vi "Drive Controller.vi"(8 "error in":errorcluster) -> ()   [LabVIEW 2020]
doc: "This VI executes continuously carrying out the current operation and responding to updates or new operation requests. It will often contain the timing or control code that is difficult to place directly in TeleOp. This VI generally opens all sensors and motors and isolates the rest of the robot code from knowing implementation details of how the operations are carried out."
uses:
  <vilib>/Rock Robotics/WPI/Framework/Completion Status.ctl
  Drive Setpoints.ctl
  Drive Operations.ctl
  <vilib>/Rock Robotics/WPI/SafetyOutput/WPI_SafetyOutputConfigMenu.ctl
  <vilib>/Rock Robotics/WPI/RobotDrive/WPI_RobotDriveOpen2MotorWithExistingMotors.vi
  <vilib>/Rock Robotics/Network Tables/NT Write Numeric Array.vi
panel:
  in  "Interactive Values":T1
  in  "Buttons":cluster{"Execute Cmd":bool, "Abort Cmd":bool}
  out "Command Timing":cluster{"Start Time (ms)":u32, "Iterations":i32}
  out "Status":T3
  out "Setpoints":T4(graph)
  out "Current\nCmd":string
  # "Tip: The graph shows the motor setpoints. It may also be helpful to observe inputs and sensor values.\nYou may also want to display tuning or debugging controls."
  # "Interactive Command: You may fill in the settings for a command\nand schedule it with the Execute button. You can observe and abort\nany command while fine tuning the code for the controller."
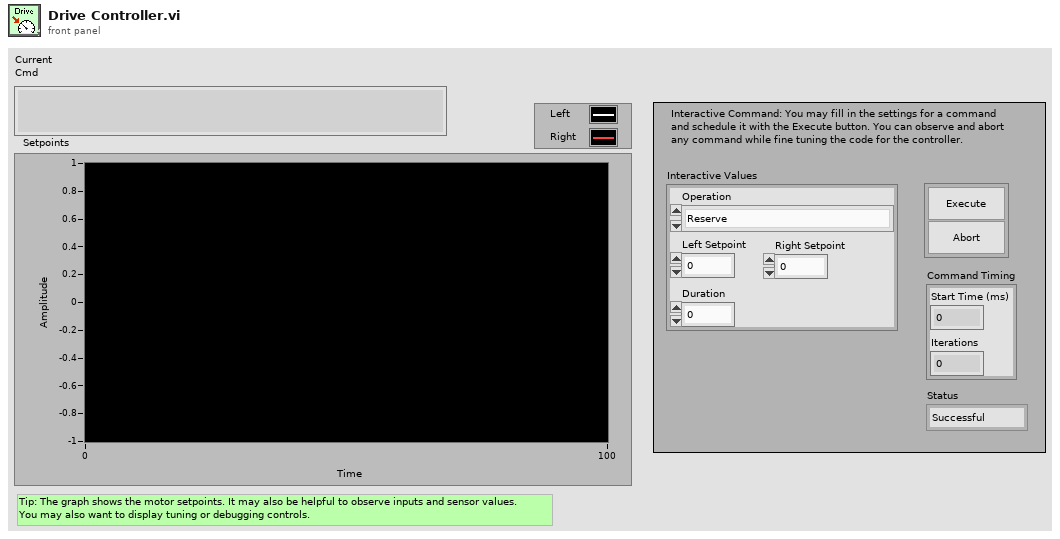
[diagram p1: front panel]
types:
  T1 = typedef "Drive Setpoints.ctl" = cluster{"Operation":T2, "Left Setpoint":dbl, "Right Setpoint":dbl, "Duration":dbl}
  T2 = typedef "Drive Operations.ctl" = enum16{"Reserve", "Read Current", "Immediate", "Drive for Time", "Drive for Distance"}
  T3 = typedef "Completion Status.ctl" = enum16{"Successful", "Aborted", "Incomplete"}
  T4 = cluster{"Left Setpoint":dbl, "Right Setpoint":dbl}
  T5 = typedef "WPI_SafetyOutputConfigMenu.ctl" = enum16{"Enable", "Disable"}
  T6 = typedef "WPI_MotorControlDeviceRef.ctl" = cluster{"DeviceStatus":errorcluster, "Type":T7, "PWM":cluster{"PWM Channel":T8, "DeadBand":T9}, "CAN":cluster{"Device Number":u8, "SetOutput VI Ref":variant, "GetOutput VI Ref":variant, "Enable VI Ref":variant, "Disable VI Ref":variant, "Data":variant}, "Invert":bool, "DIO PWM":cluster{"PWM \"Enable\" Channel":T8, "DIOChannel":T10, "PWM Rate":dbl}}
  T7 = typedef "WPI_MotorControlType.ctl" = enum16{"PWM", "CAN", "DIO PWM"}
  T8 = typedef "FPGA_DIOPWMChannel.ctl" = enum8{"PWM 0", "PWM 1", "PWM 2", "PWM 3", "PWM 4", "PWM 5", "PWM 6", "PWM 7", "PWM 8", "PWM 9", "PWM MXP 0", "PWM MXP 1", "PWM MXP 2", "PWM MXP 3", "PWM MXP 4", "PWM MXP 5", "PWM MXP 6", "PWM MXP 7", "PWM MXP 8", "PWM MXP 9", "Invalid"}
  T9 = typedef "WPI_PWMDeadband.ctl" = cluster{"Name":string, "maxPositivePwm":i32, "minPositivePwm":i32, "centerPwm":i32, "maxNegativePwm":i32, "minNegativePwm":i32, "angularRange":u16}
  T10 = typedef "FPGA_DIOChannel.ctl" = enum8{"DIO 0", "DIO 1", "DIO 2", "DIO 3", "DIO 4", "DIO 5", "DIO 6", "DIO 7", "DIO 8", "DIO 9", "DIO MXP 0", "DIO MXP 1", "DIO MXP 2", "DIO MXP 3", "DIO MXP 4", "DIO MXP 5", "DIO MXP 6", "DIO MXP 7", "DIO MXP 8", "DIO MXP 9", "DIO MXP 10", "DIO MXP 11", "DIO MXP 12", "DIO MXP 13", "DIO MXP 14", "DIO MXP 15", "SPI Port CS1", "SPI Port CS2", "SPI Port CS3", "SPI Port MISO", "SPI Port MOSI", "Invalid"}
  T11 = typedef "WPI_RobotDriveDevRef.ctl" = cluster{"DevStatus":errorcluster, "Motors[]":T6[], "Square Inputs":bool, "Max Output":dbl}
  T12 = typedef "Command Status Info.ctl" = cluster{"Name":string, "Status":T3, "notifier out":T13}
  T13 = typedef "Completion Notifier.ctl" = refnum<notifier>
  T14 = cluster{"SubSystem Data":T1, cluster{"Start Time (ms)":u32, "Iterations":i32}, cluster{"Command Info":T12, "Description":string, "Default Command":T1, "queue out":refnum<queue>, "Subsystem Name":string}}
  T15 = cluster{"SubSystem Data":T1, cluster{"Start Time (ms)":u32, "Iterations":i32}, "Default Command Arguments":cluster{"Command Info":T12, "Description":string, "Default Command":T1, "queue out":refnum<queue>, "Subsystem Name":string}}
  T16 = cluster{"Don't move motors while reserved":dbl, "Don't move motors while reserved":dbl}
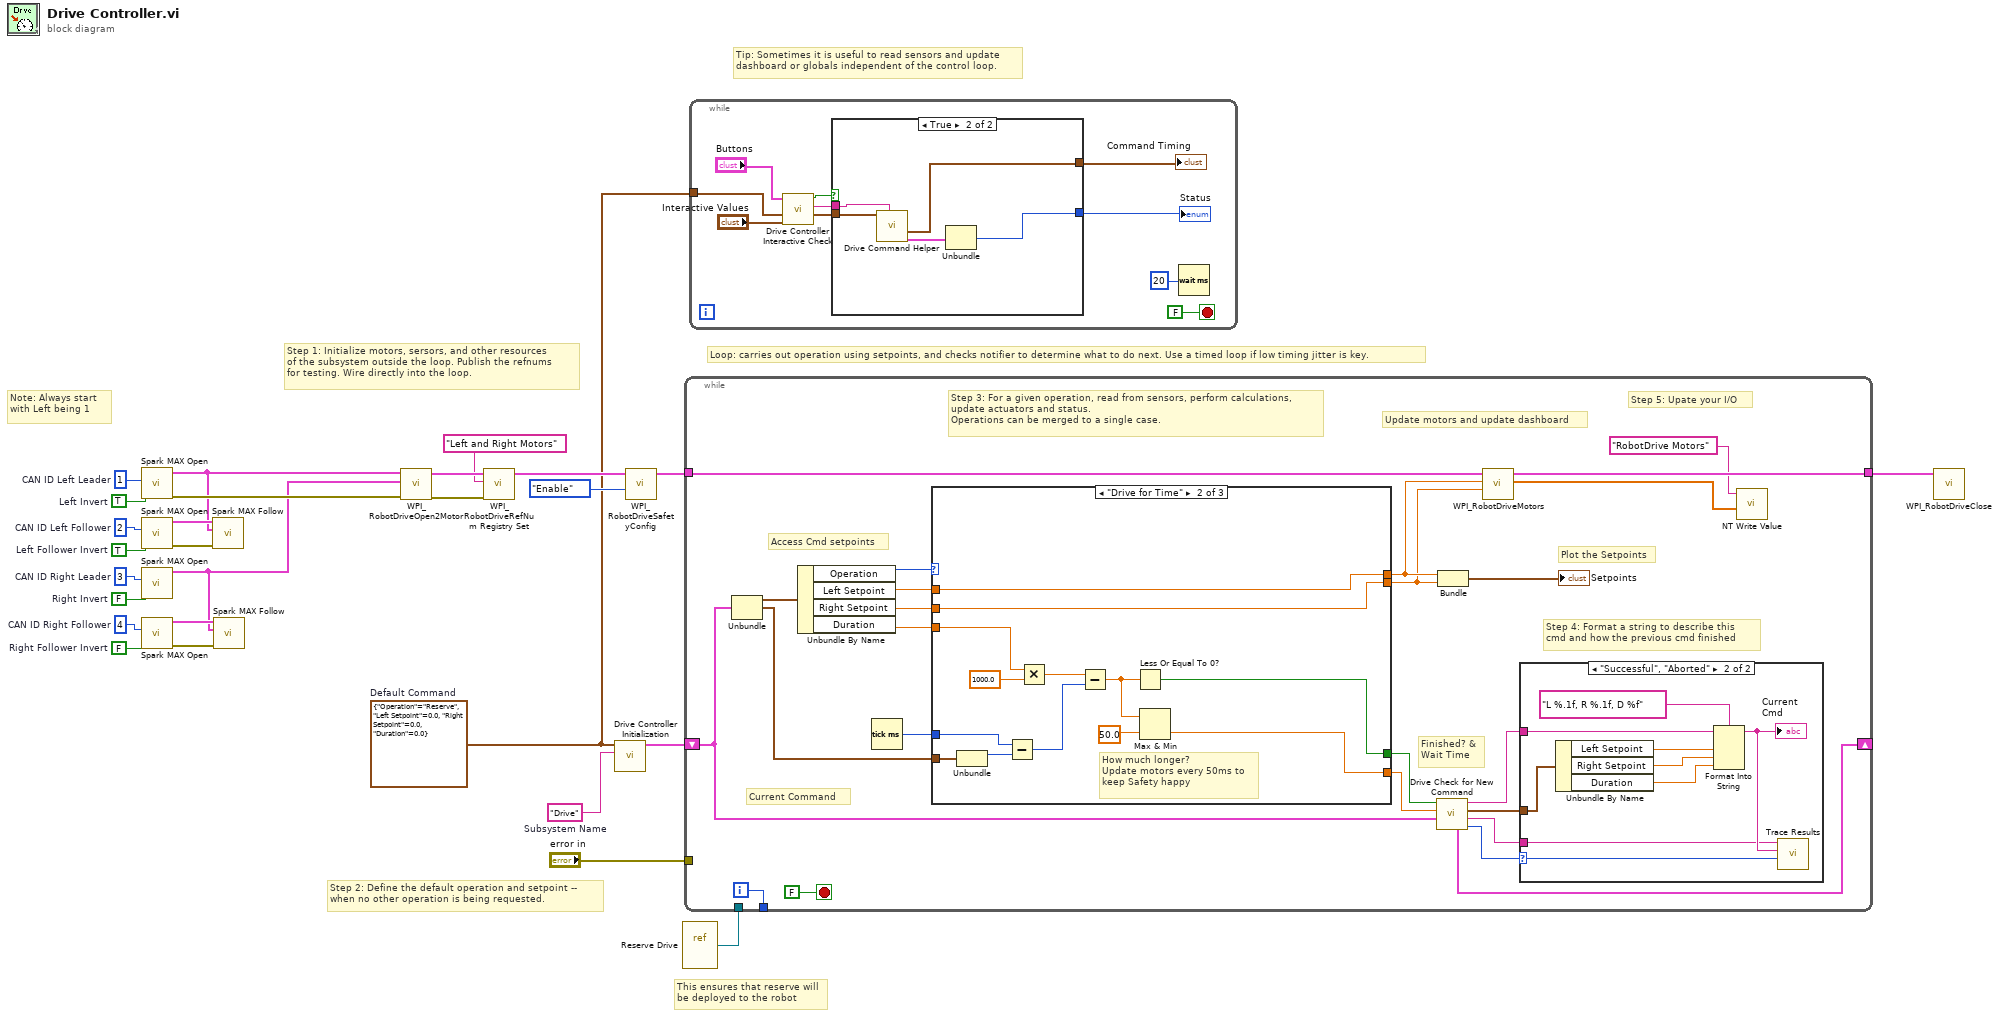
[diagram p0: block diagram]
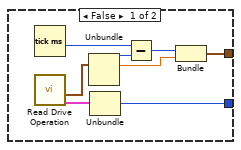
[diagram p2: hidden frame]
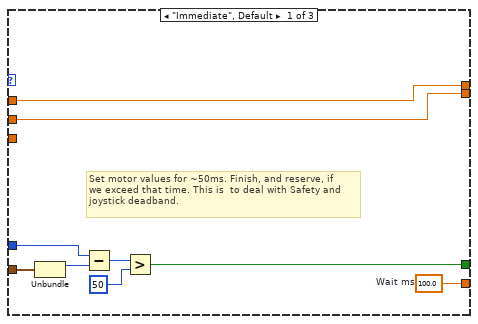
[diagram p4: hidden frame]
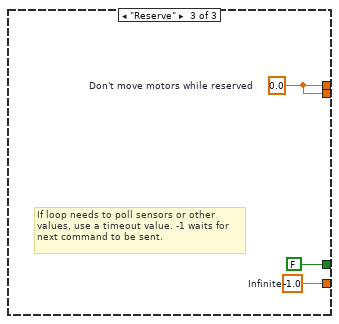
[diagram p5: hidden frame]
diagram:
  w1 = FALSE  # Right Follower Invert
  w2 = TRUE  # Left Follower Invert
  w4 = FALSE  # Right Invert
  w5 = TRUE  # Left Invert
  w6 = u8 4  # CAN ID Right Follower
  w7 = u8 3  # CAN ID Right Leader
  w8 = u8 2  # CAN ID Left Follower
  w9 = u8 1  # CAN ID Left Leader
  w17 = T1 {"Operation"=enum."Reserve", "Left Setpoint"=0.0, "Right Setpoint"=0.0, "Duration"=0.0}  # Default Command
  w27 = "Drive"  # Subsystem Name
  # "Note: Always start with Left being 1"
  # "This ensures that reserve will\nbe deployed to the robot"
  # "Tip: Sometimes it is useful to read sensors and update\ndashboard or globals independent of the control loop."
  # "Step 2: Define the default operation and setpoint --\nwhen no other operation is being requested."
  # "Step 1: Initialize motors, sersors, and other resources\nof the subsystem outside the loop. Publish the refnums\nfor testing. Wire directly into the loop."
  # "Loop: carries out operation using setpoints, and checks notifier to determine what to do next. Use a timed loop if low timing jitter is key."
  n1 = call <vilib>:"Spark MAX Open.vi"("Invert"=w5, "Device Number"=w9) -> ("error out"=w16:errorcluster, "MotorControlDeviceRef"=w11:T6)  [unwired: 8 in]
  n2 = call <vilib>:"Spark MAX Open.vi"("Invert"=w2, "Device Number"=w8) -> ("error out"=w14:errorcluster, "MotorControlDeviceRef"=w15:T6)  [unwired: 8 in]
  n3 = call <vilib>:"Spark MAX Open.vi"("Invert"=w4, "Device Number"=w7) -> ("MotorControlDeviceRef"=w10:T6)  [unwired: 8 in, 1 out]
  n4 = call <vilib>:"Spark MAX Open.vi"("Invert"=w1, "Device Number"=w6) -> ("error out"=w12:errorcluster, "MotorControlDeviceRef"=w13:T6)  [unwired: 8 in]
  n5 = call <vilib>:"Spark MAX Follow.vi"("error in (no error)"=w14, "Master Controller"=w11, "MotorControlDeviceRef"=w15) -> ()  [unwired: 7 in, 2 out]
  n6 = call <vilib>:"Spark MAX Follow.vi"("error in (no error)"=w12, "Master Controller"=w10, "MotorControlDeviceRef"=w13) -> ()  [unwired: 7 in, 2 out]
  n7 = call-poly <vilib>:"WPI_RobotDriveOpen2Motor.vi"("error in (no error)"=w16, "Right Motor Dev Ref"=w10, "Left Motor Dev Ref"=w11) -> ("error out"=w24:errorcluster, "RobotDriveDevRef"=w26:T11)  [unwired: 2 in, 5 out]
  n8 = call <vilib>:"WPI_RobotDriveRefNum Registry Set.vi"("error in (no error)"=w24, "refnum name"="Left and Right Motors", "RobotDriveDevRef"=w26) -> ("RobotDriveDevRef"=w23:T11)  [unwired: 1 in, 7 out]
  n9 = call "Drive Controller Initialization.vi"("Subsystem Name"=w27, "Default Command"=w17) -> ("Current Command"=w19:T14)  [unwired: 9 in]
  n10 = call <vilib>:"WPI_RobotDriveSafetyConfig.vi"("mode"=WPI_SafetyOutputConfigMenu."Enable", "RobotDriveDevRef"=w23) -> ("RobotDriveDevRef"=w21:T11)  [unwired: 8 in, 1 out]
  n11 = vi-ref "Reserve Drive.vi"() -> (w18:refnum<vi>)
  n12 = while {
    shift-right: [w38] -> _
    shift-left: w19 -> [w31]
    tunnel: [w50] -> _
    tunnel: w21 -> [w46]
    tunnel: "error in" -> [_]
    tunnel: w18 -> [_]
    tunnel: [w30] -> w3
    i -> [w50]
    stop <- FALSE stop-if-true
    # "Step 5: Upate your I/O"
    # "Step 4: Format a string to describe this\ncmd and how the previous cmd finished"
    # "Current Command"
    # "Update motors and update dashboard"
    # "Plot the Setpoints"
    # "Access Cmd setpoints"
    # "Finished? &\nWait Time"
    # "Step 3: For a given operation, read from sensors, perform calculations,\nupdate actuators and status.\nOperations can be merged to a single case."
    n13 = Unbundle(w31) -> ("SubSystem Data"=w45:T1, w32:cluster{"Start Time (ms)":u32, "Iterations":i32})  [unwired: 1 out]
    n14 = Unbundle By Name(w45) -> ("Operation"=w44:T2, "Left Setpoint"=w43:dbl, "Right Setpoint"=w42:dbl, "Duration"=w41:dbl)
    n15 = Tick Count (ms)() -> (millisecond timer value=w40:u32)
    n16 = case shown="\"Drive for Time\"" w44 {
      tunnel: [w69 w70 w85] -> w37
      tunnel: [w62 w77 FALSE ("ignore previous (F)")] -> w36
      tunnel: w32 -> [w61 w79 _]
      tunnel: [w68 w76 w83] -> w48
      tunnel: [w67 w75 w83] -> w47
      tunnel: w43 -> [w68 w76 _]
      tunnel: w42 -> [w67 w75 _]
      tunnel: w41 -> [_ w74 _]
      tunnel: w40 -> [w63 w73 _]
      frame "Immediate", Default {
        w69 = 100.0  # Wait ms
        # "Set motor values for ~50ms. Finish, and reserve, if\nwe exceed that time. This is  to deal with Safety and\njoystick deadband."
        n17 = Unbundle(w61) -> ("Start Time (ms)"=w64:u32)  [unwired: 1 out]
        n18 = Subtract(x=w63, y=w64) -> (x-y=w65:u32)
        n19 = Greater?(x=w65, y=u8 50 ("Left Motor")) -> (0:w62:bool)
      }
      frame "Drive for Time" {
        # "How much longer?\nUpdate motors every 50ms to\nkeep Safety happy"
        n20 = Unbundle(w79) -> ("Start Time (ms)"=w78:u32)  [unwired: 1 out]
        n21 = Subtract(x=w73, y=w78) -> (x-y=w82:u32)
        n22 = Multiply(x=w74, y=1000.0) -> (x*y=w81:dbl)
        n23 = Subtract(x=w81, y=w82) -> (x-y=w72:dbl)
        n24 = Less Or Equal To 0?(x=w72) -> (x <= 0?=w77:bool)
        n25 = Max & Min(x=w72, y=50.0) -> (min(x,y)=w70:dbl)  [unwired: 1 out]
      }
      frame "Reserve" {
        w83 = 0.0  # Don't move motors while reserved
        w85 = -1.0  # Infinite
        # "If loop needs to poll sensors or other\nvalues, use a timeout value. -1 waits for\nnext command to be sent."
      }
    }
    n26 = call "Drive Check for New Command.vi"("input cluster"=w31, "Wait time (ms)"=w37, "Finished?"=w36) -> ("Completion"=w39:T3, "Subsystem Name"=w33:string, "Current Command"=w34:T1, "Initial Trace String"=w35:string, "Next Command"=w38:T15)  [unwired: 4 in]
    n27 = Bundle("Don't move motors while reserved"=w48, "Don't move motors while reserved"=w47) -> (→"Setpoints":T16)  [unwired: 1 in]
    n28 = call <vilib>:"WPI_RobotDriveMotors.vi"("RightSpeed"=w47, "LeftSpeed"=w48, "RobotDriveDevRef"=w46) -> ("Motor Values"=w29:dbl[], "RobotDriveDevRef"=w30:T11)  [unwired: 1 in, 6 out]
    n29 = case shown="\"Successful\", \"Aborted\"" w39 {
      selector: w39 -> [_ w60]
      tunnel: w35 -> [_ w55]
      tunnel: w34 -> [_ w56]
      tunnel: w33 -> [_ w52]
      frame "Incomplete", Default {
        # "Continuing current command"
      }
      frame "Successful", "Aborted" {
        # "Report and setup for next command"
        n30 = Unbundle By Name(w56) -> ("Left Setpoint"=w58:dbl, "Right Setpoint"=w59:dbl, "Duration"=w53:dbl)
        n31 = Format Into String(format string="L %.1f, R %.1f, D %f", initial string=w55, w58, w59, w53) -> (resulting string=w54:string)  [unwired: 1 in, 1 out]
        "Current\nCmd" <- w54
        n32 = call <vilib>:"Trace Results.vi"("Status of previous command"=w60, "Description"=w54, "Subsystem"=w52) -> ()  [unwired: 9 in]
      }
    }
    n33 = call-poly <vilib>:"NT Write Value.vi"("Numeric Array"=w29, "Name"="RobotDrive Motors") -> ()  [unwired: 9 in, 1 out]
  }
  n34 = while {
    tunnel: w17 -> [w87]
    stop <- FALSE stop-if-true
    n35 = call "Drive Controller Interactive Check.vi"("Interactive Command In"="Interactive Values", "Default Command"=w87, "Buttons"="Buttons") -> ("Interactive Command Out"=w89:T1, "Trace String"=w90:string, "Schedule"=w91:bool)  [unwired: 6 in]
    n36 = case shown="True" w91 {
      tunnel: [w100 w108] -> w92
      tunnel: [w99 w104] -> w93
      tunnel: w90 -> [_ w106]
      tunnel: w89 -> [_ w105]
      frame False {
        n37 = Tick Count (ms)() -> (millisecond timer value=w103:u32)
        n38 = call "Read Drive Operation.vi"() -> ("Command Info"=w97:T12, "SubSystem Data"=w96:T1)  [unwired: 9 in, 1 out]
        n39 = Unbundle(w96) -> ("Operation"=w101:T2, "Left Setpoint"=w98:dbl)  [unwired: 2 out]
        n40 = Unbundle(w97) -> ("Status"=w100:T3)  [unwired: 2 out]
        n41 = Subtract(x=w103, y=w101) -> (x-y=w102:u32)
        n42 = Bundle(w102, "Left Setpoint"=w98) -> (w99:cluster{u32, "Left Setpoint":dbl})  [unwired: 1 in]
      }
      frame True {
        n43 = call "Drive Command Helper.vi"("Description"=w106, "SubSystem Data"=w105) -> ("Command Info Out"=w107:T12, "Command Timing"=w104:cluster{"Start Time (ms)":u32, "Iterations":i32})  [unwired: 7 in, 1 out]
        n44 = Unbundle(w107) -> ("Status"=w108:T3)  [unwired: 2 out]
      }
    }
    "Status" <- w92
    "Command Timing" <- w93
    n45 = Wait (ms)(milliseconds to wait=u32 20) -> ()  [unwired: 1 out]
  }
  n46 = call <vilib>:"WPI_RobotDriveClose.vi"("RobotDriveDevRef"=w3) -> ()  [unwired: 10 in, 1 out]
